vi "Motor Init.vi"(4 "Brake / Coast Mode":T8, 5 "I":dbl, 6 "D":dbl, 7 "P":dbl, 8 "error in (no error)":errorcluster, 9 "Invert":bool, 10 "Encoder Codes Per Rev":u16=64, 11 "Device Number":u8) -> (0 "error out":errorcluster, 3 "CAN Jaguar Ref Out":T1={"DeviceStatus"={"status"=FALSE, "code"=0, "source"=""}, "Type"=enum."PWM", "PWM"={"Digital Module"=enum."Digital Module 2", "PWM Channel"=enum."PWM 1", "DeadBand"={"Name"="", "maxPositivePwm"=0, "minPositivePwm"=0, "centerPwm"=0, "maxNegativePwm"=0, "minNegativePwm"=0, "angularRange"=0}}, "CAN"={"Device Number"=0, "Control Mode"=enum."Percent VBus", "Semaphore"=refnum, "Max Vout"=12.0}, "Invert"=FALSE, "TransformRef"=refnum, "InvTransformRef"=refnum})   [LabVIEW 2012]
uses:
  <vilib>/Rock Robotics/WPI/CAN/Jaguar/SubVIs/WPI_CANJaguar_BrakeCoastMode.ctl
  <vilib>/Rock Robotics/WPI/MotorControl/WPI_MotorControlDeviceRef.ctl
  <vilib>/Rock Robotics/SystemInterfaces/Typedef/FPGA_TypedefDigitalModule.ctl
  <vilib>/Rock Robotics/SystemInterfaces/DIO/FPGA_DIOPWMChannel.ctl
  <vilib>/Rock Robotics/WPI/PWM/WPI_PWMDeadband.ctl
  <vilib>/Rock Robotics/WPI/CAN/Jaguar/SubVIs/WPI_CANJaguar_ControlMode.ctl
  <vilib>/Rock Robotics/WPI/PWM/WPI_PWMTransform_ConPane.ctl
  <vilib>/Rock Robotics/WPI/CAN/Jaguar/SubVIs/WPI_CANJaguar_SpeedReference.ctl
  <vilib>/Rock Robotics/WPI/MotorControl/WPI_MotorControlOpenCANJaguar.vi
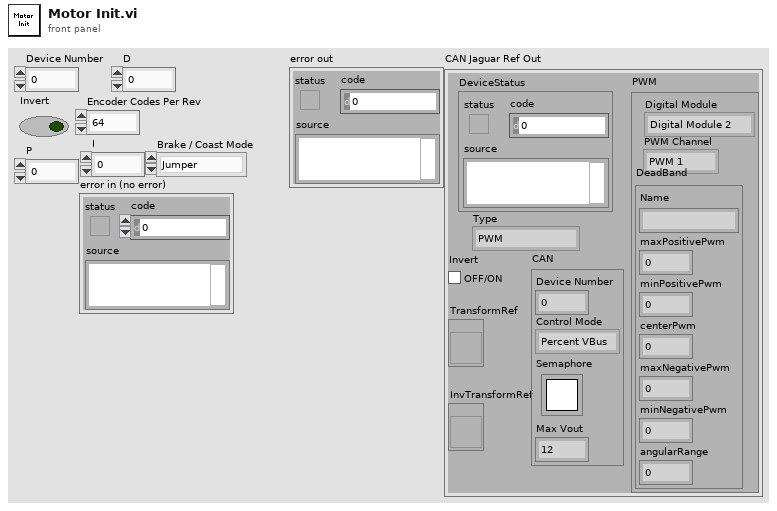
[diagram p1: front panel]
types:
  T1 = typedef "WPI_MotorControlDeviceRef.ctl" = cluster{"DeviceStatus":errorcluster, "Type":enum16{"PWM", "CAN"}, "PWM":cluster{"Digital Module":T2, "PWM Channel":T3, "DeadBand":T4}, "CAN":cluster{"Device Number":u8, "Control Mode":T5, "Semaphore":T6, "Max Vout":dbl}, "Invert":bool, "TransformRef":T7, "InvTransformRef":T7}
  T2 = typedef "FPGA_TypedefDigitalModule.ctl" = enum16{"Digital Module 1", "Digital Module 2"}
  T3 = typedef "FPGA_DIOPWMChannel.ctl" = enum8{"PWM 1", "PWM 2", "PWM 3", "PWM 4", "PWM 5", "PWM 6", "PWM 7", "PWM 8", "PWM 9", "PWM 10", "Invalid"}
  T4 = typedef "WPI_PWMDeadband.ctl" = cluster{"Name":string, "maxPositivePwm":i32, "minPositivePwm":i32, "centerPwm":i32, "maxNegativePwm":i32, "minNegativePwm":i32, "angularRange":u16}
  T5 = typedef "WPI_CANJaguar_ControlMode.ctl" = enum8{"Percent VBus", "Current", "Speed", "Position", "Voltage"}
  T6 = typedef "Semaphore RefNum" = refnum<k1>
  T7 = typedef "WPI_PWMTransform_ConPane.ctl" = refnum<vi>
  T8 = typedef "WPI_CANJaguar_BrakeCoastMode.ctl" = enum8{"Jumper", "Brake", "Coast"}
  T9 = typedef "WPI_CANJaguar_SpeedReference.ctl" = u8
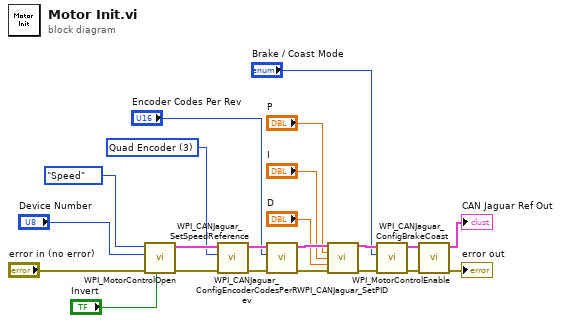
[diagram p0: block diagram]
diagram:
  w17 = T9 3 items=["Encoder"=0, "Inv Encoder"=2, "Quad Encoder"=3, "None"=255] ("Speed Reference")
  n1 = call-poly <vilib>:"WPI_MotorControlOpen.vi"("Invert"="Invert", "error in (no error)"="error in (no error)", "Device Number"="Device Number", "Control Mode"=WPI_CANJaguar_ControlMode."Speed") -> ("error out"=w19:errorcluster, "MotorControlDeviceRef"=w18:T1)  [unwired: 6 in]
  n2 = call <vilib>:"WPI_CANJaguar_SetSpeedReference.vi"("error in (no error)"=w19, "Speed Reference"=w17, "CAN Jaguar Ref"=w18) -> ("error out"=w16:errorcluster, "CAN Jaguar Ref Out"=w15:T1)  [unwired: 7 in]
  n3 = call <vilib>:"WPI_CANJaguar_ConfigEncoderCodesPerRev.vi"("error in (no error)"=w16, "Encoder Codes Per Rev"="Encoder Codes Per Rev", "CAN Jaguar Ref"=w15) -> ("error out"=w12:errorcluster, "CAN Jaguar Ref Out"=w13:T1)  [unwired: 7 in]
  n4 = call <vilib>:"WPI_CANJaguar_SetPID.vi"("CAN Jaguar Ref"=w13, "P"="P", "I"="I", "D"="D", "error in (no error)"=w12) -> ("CAN Jaguar Ref Out"=w7:T1, "error out"=w8:errorcluster)  [unwired: 9 in]
  n5 = call <vilib>:"WPI_CANJaguar_ConfigBrakeCoast.vi"("error in (no error)"=w8, "Brake / Coast Mode"="Brake / Coast Mode", "CAN Jaguar Ref"=w7) -> ("error out"=w3:errorcluster, "CAN Jaguar Ref Out"=w4:T1)  [unwired: 7 in]
  n6 = call <vilib>:"WPI_MotorControlEnable.vi"("error in (no error)"=w3, "CAN Jaguar Ref"=w4) -> ("error out"=→"error out":errorcluster, "CAN Jaguar Ref Out"=→"CAN Jaguar Ref Out":T1)  [unwired: 8 in]
